vi "Send Engine Pointer to Async Threads.vi"(8 "error in (no error)":errorcluster, 11 "Framework in":refnum<class "Framework.lvclass">) -> (0 "error out":errorcluster, 3 "Framework out":refnum<class "Framework.lvclass">)   [LabVIEW 2017, in "DSF Core.lvlib" / "Framework.lvclass"]
uses:
  Framework.lvclass
  Framework.lvclass/Framework.ctl
  Buffer/Buffers.lvclass/Buffers.ctl
  Interfaces/Dispatcher/Inline Buffer Parameters.ctl
  <vilib>/NI/Memory Manager/Classes/Pointer/Pointer.lvclass/Pointer.ctl
  Buffer/Buffer.lvclass
  C:/Program Files (x86)/National Instruments/LabVIEW 2017/vi.lib/NI/Memory Manager/Classes/Pointer/Pointer.lvclass
  Thread/Plugin/Plugin Thread.lvclass
  Plugin/Plugin.lvclass
  Buffer/Buffers.lvclass
  <vilib>/NI/Memory Manager/Classes/Pointer/Pointer.lvclass
  Interfaces/Dispatcher/Dispatcher Interface.lvclass
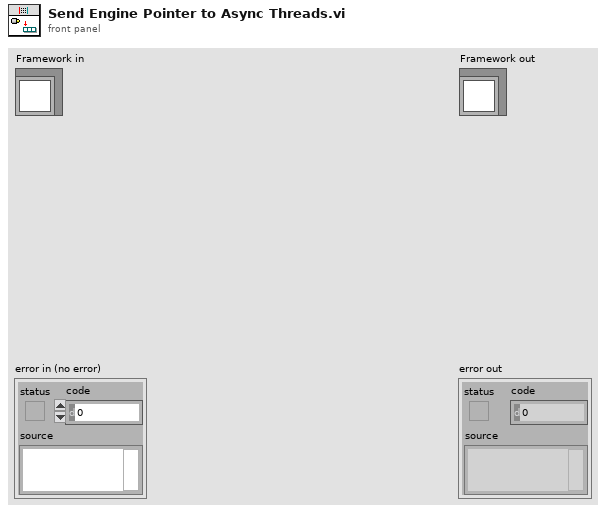
[diagram p1: front panel]
types:
  T1 = typedef "DSF Core.lvlib/Dispatcher Interface.lvclass/Inline Buffer Parameters.ctl" = cluster{"address":u64, "size":u64}
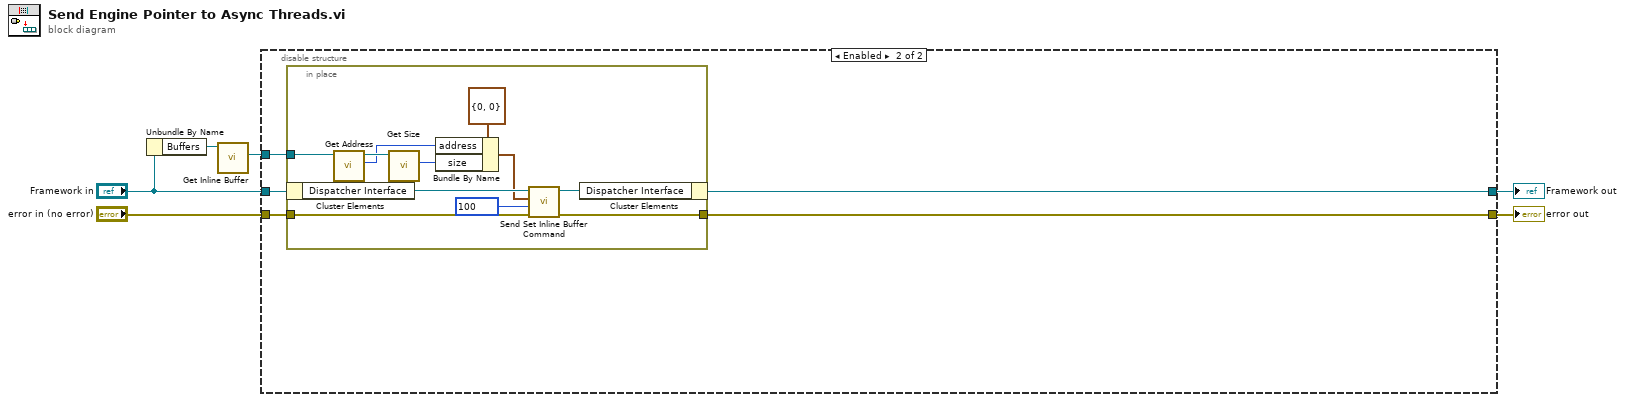
[diagram p0: block diagram]
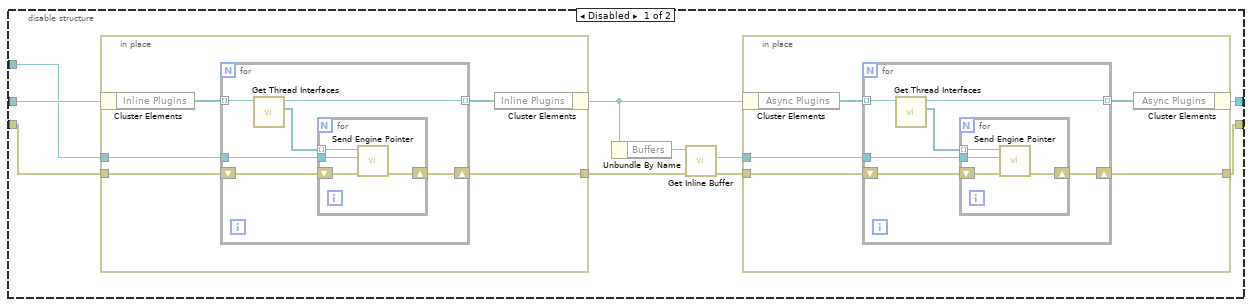
[diagram p2: hidden frame]
diagram:
  n1 = Unbundle By Name("Framework in") -> ("Buffers"=w2:refnum<class "Buffers.lvclass">)
  n2 = call "Get Inline Buffer.vi"("Buffers in"=w2) -> ("Inline Buffer"=w1:refnum<class "Buffer.lvclass">)  [unwired: 9 in, 1 out]
  n3 = disable-structure shown="Enabled" {
    disable-tunnel: [w15 w47] -> w6
    disable-tunnel: [w14 w46] -> w5
    disable-tunnel: "error in (no error)" -> [w13 w48]
    disable-tunnel: "Framework in" -> [w11 w50]
    disable-tunnel: w1 -> [w10 w49]
    frame Disabled {
      n4 = in-place {
        in-place-border: w13 -> [w18]
        in-place-border: [w17] -> w12
        in-place-border: w10 -> [w16]
        n5 = in-place-cluster #1(w11) -> ("Inline Plugins"=w20:refnum<class "Plugin.lvclass">[])
        n6 = for {
          tunnel: w20 -> [w26] mode=indexing
          tunnel: [w25] -> w19 mode=indexing
          shift-right: [w23] -> w17
          shift-left: w18 -> [w22]
          tunnel: w16 -> [w21]
          n7 = call "Get Thread Interfaces.vi"("Plugin in"=w26) -> ("Plugin Interfaces"=w24:refnum<class "Plugin Interface.lvclass">[], "Plugin out"=w25:refnum<class "Plugin.lvclass">)  [unwired: 9 in]
          n8 = for {
            tunnel: w24 -> [w30] mode=indexing
            shift-right: [w29] -> w23
            shift-left: w22 -> [w28]
            tunnel: w21 -> [w27]
            n9 = call "Send Engine Pointer.vi"("error in (no error)"=w28, "Framework Inline Buffer"=w27, "Plugin Interface in"=w30) -> ("error out"=w29:errorcluster)  [unwired: 7 in, 1 out]
          }
        }
        n10 = in-place-cluster #1("Inline Plugins"=w19) -> (w8:refnum<class "Framework.lvclass">)
      }
      n11 = Unbundle By Name(w8) -> ("Buffers"=w9:refnum<class "Buffers.lvclass">)
      n12 = call "Get Inline Buffer.vi"("Buffers in"=w9) -> ("Inline Buffer"=w7:refnum<class "Buffer.lvclass">)  [unwired: 9 in, 1 out]
      n13 = in-place {
        in-place-border: w12 -> [w33]
        in-place-border: [w32] -> w14
        in-place-border: w7 -> [w31]
        n14 = in-place-cluster #2(w8) -> ("Async Plugins"=w35:refnum<class "Plugin.lvclass">[])
        n15 = for {
          tunnel: w35 -> [w41] mode=indexing
          tunnel: [w40] -> w34 mode=indexing
          shift-right: [w38] -> w32
          shift-left: w33 -> [w37]
          tunnel: w31 -> [w36]
          n16 = call "Get Thread Interfaces.vi"("Plugin in"=w41) -> ("Plugin Interfaces"=w39:refnum<class "Plugin Interface.lvclass">[], "Plugin out"=w40:refnum<class "Plugin.lvclass">)  [unwired: 9 in]
          n17 = for {
            tunnel: w39 -> [w45] mode=indexing
            shift-right: [w44] -> w38
            shift-left: w37 -> [w43]
            tunnel: w36 -> [w42]
            n18 = call "Send Engine Pointer.vi"("error in (no error)"=w43, "Framework Inline Buffer"=w42, "Plugin Interface in"=w45) -> ("error out"=w44:errorcluster)  [unwired: 7 in, 1 out]
          }
        }
        n19 = in-place-cluster #2("Async Plugins"=w34) -> (w15:refnum<class "Framework.lvclass">)
      }
    }
    frame Enabled {
      n20 = in-place {
        in-place-border: w49 -> [w61]
        in-place-border: w48 -> [w57]
        in-place-border: [w56] -> w46
        n21 = in-place-cluster #3(w50) -> ("Dispatcher Interface"=w59:refnum<class "Dispatcher Interface.lvclass">)
        n22 = call <vilib>:"Get Address.vi"("Pointer in"=w61) -> ("address"=w53:u64, "Pointer out"=w60:refnum<class "Buffer.lvclass">)  [unwired: 9 in]
        n23 = call <vilib>:"Get Size.vi"("Pointer in"=w60) -> ("size"=w54:u64)  [unwired: 9 in, 1 out]
        n24 = Bundle By Name(cluster=T1 {"address"=0, "size"=0} ("Inline Buffer Parameters"), "address"=w53, "size"=w54) -> (w52:T1)
        n25 = call "Send Set Inline Buffer Command.vi"("error in (no error)"=w57, "timeout in ms (0)"=100, "Inline Buffer Parameters"=w52, "Dispatcher Interface in"=w59) -> ("error out"=w56:errorcluster, "Dispatcher Interface out"=w58:refnum<class "Dispatcher Interface.lvclass">)  [unwired: 5 in, 1 out]
        n26 = in-place-cluster #3("Dispatcher Interface"=w58) -> (w47:refnum<class "Framework.lvclass">)
      }
    }
  }
  "error out" <- w5
  "Framework out" <- w6
